vi "Prompt for Step--Check for Input.vi"(7 "Control Ref Map":map{string, refnum<vi>}(c390), 8 "error in (no error)":errorcluster, 9 "Macro Hotkey":T1(array[ring]), 10 "Keyboard Ref":refnum<k1>, 11 "Mouse Action in":refnum<class "Mouse Action.lvclass">) -> (0 "error out":errorcluster, 3 "Mouse Action out":refnum<class "Mouse Action.lvclass">)   [LabVIEW 2020, in "MacroAssert.lvlib" / "Mouse Action.lvclass"]
uses:
  Mouse Action.lvclass
  Mouse Action Type.ctl
  Mouse Action.lvclass/Mouse Action.ctl
  Support/Get Control Reference by Label (0D STR).vi
  MacroAssert.lvlib
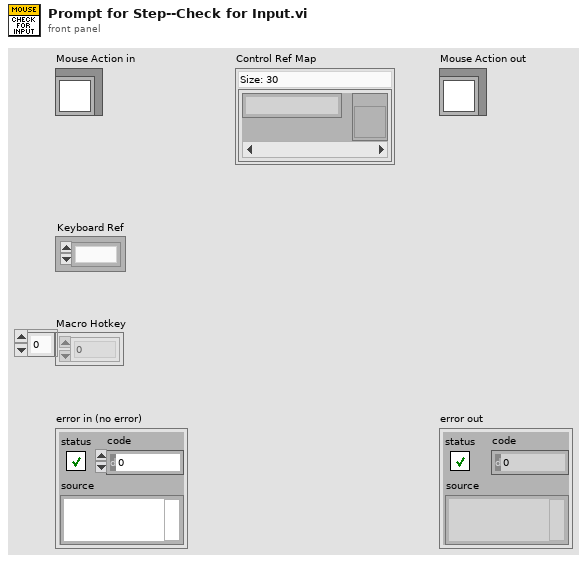
[diagram p1: front panel]
types:
  T1 = enum16{"0", "1", "2", "3", "4", "5", "6", "7", "8", "9", "A", "B", "C", "D", "E", "F", "G", "H", "I", "J", "K", "L", "M", "N", "O", "P", "Q", "R", "S", "T", "U", "V", "W", "X", "Y", "Z", "F1", "F2", "F3", "F4", "F5", "F6", "F7", "F8", "F9", "F10", "F11", "F12", "F13", "F14", "F15", "ADD", "BACK", "BACKSLASH", "CAPITAL", "COMMA", "DECIMAL", "DELETE", "DIVIDE", "DOWN", "END", "EQUALS", "ESCAPE", "GRAVE (`)", "HOME", "INSERT", "LBRACKET", "LCONTROL", "LEFT", "L ALT", "LSHIFT", "LWIN", "MINUS", "MULTIPLY", "NEXT", "NUMLOCK", "NUMPAD_0", "NUMPAD_1", "NUMPAD_2", "NUMPAD_3", "NUMPAD_4", "NUMPAD_5", "NUMPAD_6", "NUMPAD_7", "NUMPAD_8", "NUMPAD_9", "PAUSE", "PERIOD", "PRIOR (PG UP)", "RBRACKET", "RCONTROL", "RETURN", "RIGHT", "R ALT", "RSHIFT", "RWIN", "SCROLL", "SEMICOLON", "SLASH", "SPACE", "SUBTRACT", "TAB", "UP", "ENTER (num pad)", "' (quote)"}[]
  T2 = typedef "MacroAssert.lvlib/Mouse Action.lvclass/Mouse Action Type.ctl" = enum16{"Click", "Absolute Move", "Absolute Move and Click", "Relative Move", "Relative Move and Click", "Wheel Up", "Wheel Down"}
  T3 = typedef "MacroAssert.lvlib/Mouse Action.lvclass/Relative Movement Type.ctl" = enum16{"Pixels from Current Position", "Pixels from Top-Left of Control", "Pixels from Top-Left of Window", "Percentage from Top-Left of Control", "Percentage from Top-Left of Window", "Percentage from Top-Left of Screen"}
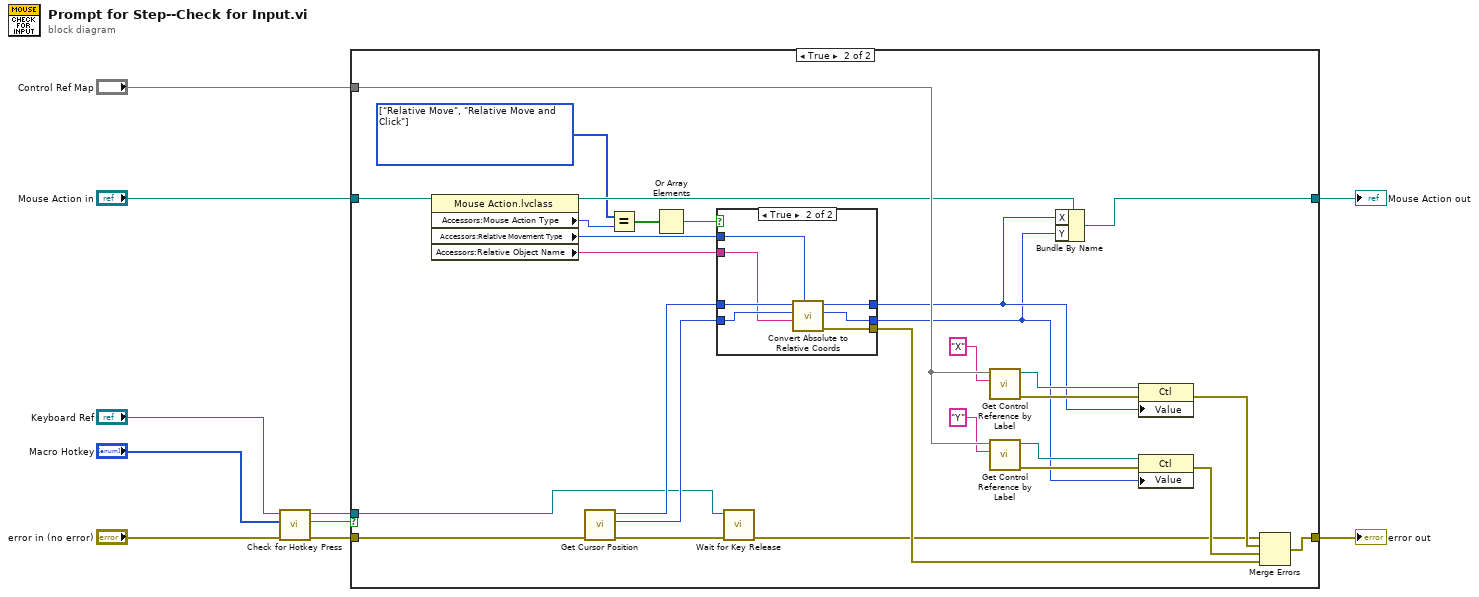
[diagram p0: block diagram]
diagram:
  n1 = call "Check for Hotkey Press.vi"("error in (no error)"="error in (no error)", "Hotkey"="Macro Hotkey", "Keyboard"="Keyboard Ref") -> ("error out"=w9:errorcluster, "Pressed?"=w3:bool, "Keyboard out"=w1:refnum<k1>)  [unwired: 6 in]
  n2 = case shown="True" w3 {
    tunnel: "Mouse Action in" -> [w11 w36]
    tunnel: [w11 w35] -> w5
    tunnel: "Control Ref Map" -> [_ w31]
    tunnel: w9 -> [w12 w16]
    tunnel: [w12 w40] -> w8
    tunnel: w1 -> [_ w13]
    frame False {
    }
    frame True {
      w26 = T2[] [enum."Relative Move", enum."Relative Move and Click"] items=["Click", "Absolute Move", "Absolute Move and Click", "Relative Move", "Relative Move and Click", "Wheel Up", "Wheel Down"]
      n3 = property class="Mouse Action.lvclass"(reference=w36) -> (reference out=w28:refnum<class "Mouse Action.lvclass">, "Accessors:Mouse Action Type"=w27:T2, "Accessors:Relative Movement Type"=w23:T3, "Accessors:Relative Object Name"=w22:string)  [unwired: 1 in, 1 out]
      n4 = call "Get Cursor Position.vi"("error in (no error)"=w16) -> ("error out"=w15:errorcluster, "Y"=w17:i32, "X"=w18:i32)  [unwired: 8 in]
      n5 = Equal?(x=w26, y=w27) -> (x = y?=w25:bool[])
      n6 = Or Array Elements(Boolean array=w25) -> (logical OR=w24:bool)
      n7 = case shown="True" w24 {
        tunnel: w18 -> [w41 w49]
        tunnel: w17 -> [w42 w48]
        tunnel: w23 -> [_ w47]
        tunnel: w22 -> [_ w46]
        tunnel: [w41 w45] -> w21
        tunnel: [w42 w44] -> w20
        tunnel: [_ w43] -> w19
        frame False {
        }
        frame True {
          n8 = call "Convert Absolute to Relative Coords.vi"("Relative Movement Type"=w47, "Relative Object Name"=w46, "Y"=w48, "X"=w49) -> ("error out"=w43:errorcluster, "Relative Y"=w44:i32, "Relative X"=w45:i32)  [unwired: 5 in]
        }
      }
      n9 = call "Wait for Key Release.vi"("error in (no error)"=w15, "Keyboard"=w13) -> ("error out"=w14:errorcluster)  [unwired: 8 in, 1 out]
      n10 = call-poly "Get Control Reference by Label.vi"("Control Name"="X", "Control Ref Map"=w31) -> ("error out"=w34:errorcluster, "Control Ref"=w32:refnum<vi>)  [unwired: 7 in, 1 out]
      n11 = call-poly "Get Control Reference by Label.vi"("Control Name"="Y", "Control Ref Map"=w31) -> ("error out"=w37:errorcluster, "Control Ref"=w33:refnum<vi>)  [unwired: 7 in, 1 out]
      n12 = Bundle By Name(cluster=w28, "X"=w21, "Y"=w20) -> (w35:refnum<class "Mouse Action.lvclass">)
      n13 = property class="Ctl"(reference=w32, error in=w34, "Value"=w21) -> (error out=w38:errorcluster)  [unwired: 1 out]
      n14 = property class="Ctl"(reference=w33, error in=w37, "Value"=w20) -> (error out=w39:errorcluster)  [unwired: 1 out]
      n15 = Merge Errors(w14, w38, w39, w19) -> (w40:errorcluster)
    }
  }
  "error out" <- w8
  "Mouse Action out" <- w5
